vi "Run_Core.vi"(0 "For Loop in":refnum<class "For Loop.lvclass">, 11 "error in (no error)":errorcluster) -> (4 "For Loop out":refnum<class "For Loop.lvclass">, 6 "Return":variant, 15 "error out":errorcluster)   [LabVIEW 2016, in "For Loop.lvclass"]
uses:
  For Loop.lvclass
  D:/TOOLS/LabVIEW-Script-Language.git/trunk/source code/LSL components/functions/functionsbase/functionbase.lvclass
  functionsbase/functionbase.lvclass/functionbase.ctl
  For Loop.lvclass/For Loop.ctl
  functionsbase/properties/Read Smart Syntax Representation.vi
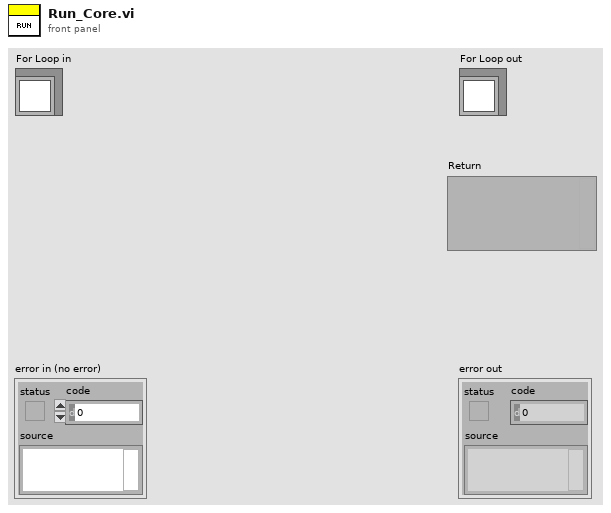
[diagram p1: front panel]
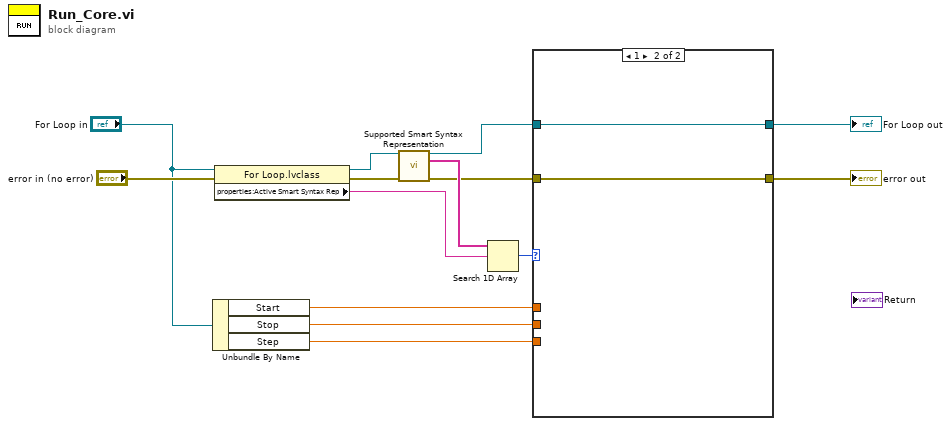
[diagram p0: block diagram]
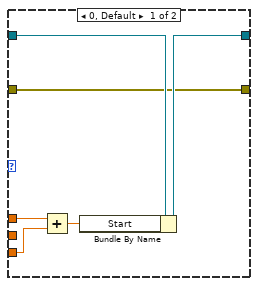
[diagram p2: hidden frame]
diagram:
  n1 = Unbundle By Name("For Loop in") -> ("Start"=w7:dbl, "Stop"=w6:dbl, "Step"=w5:dbl)
  n2 = property class="For Loop.lvclass"(reference="For Loop in", error in="error in (no error)") -> (reference out=w10:refnum<class "For Loop.lvclass">, error out=w13:errorcluster, "properties:Active Smart Syntax Rep"=w8:string)
  n3 = call-dynamic "Supported Smart Syntax Representation.vi"("For Loop in"=w10, "error in (no error)"=w13) -> ("For Loop out"=w4:refnum<class "For Loop.lvclass">, "Smart Syntax Representation List"=w12:string[], "error out"=w2:errorcluster)  [unwired: 11 in]
  n4 = Search 1D Array(1D array=w12, element=w8) -> (index of element=w11:i32)  [unwired: 1 in]
  n5 = case shown="1" w11 {
    tunnel: w7 -> [w19 _]
    tunnel: w6 -> [_ _]
    tunnel: w5 -> [w18 _]
    tunnel: w4 -> [w20 w22]
    tunnel: [w16 w22] -> w3
    tunnel: w2 -> [w15 w21]
    tunnel: [w15 w21] -> w1
    frame 0, Default {
      n6 = Add(x=w19, y=w18) -> (x+y=w17:dbl)
      n7 = Bundle By Name(cluster=w20, "Start"=w17) -> (w16:refnum<class "For Loop.lvclass">)
    }
    frame 1 {
    }
  }
  "error out" <- w1
  "For Loop out" <- w3
